vi "index_trigger.vi"(10 "fifo-counter":i32) -> (2 "index trigger":bool)   [LabVIEW 2015]
panel:
  # "(Ignoring the first iteration) This subvi returns true when the previous value \npassed in does not equal the current value passed in."
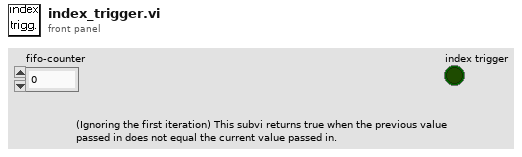
[diagram p1: front panel]
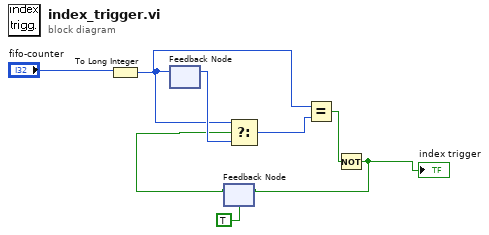
[diagram p0: block diagram]
diagram:
  n1 = To Long Integer(number="fifo-counter") -> (32bit integer=w6:i32)
  n2 = feedback #1() -> (w8:i32)  [unwired: 1 in]
  n3 = feedback-in #1(w6) -> ()
  n4 = feedback #2(TRUE) -> (w4:bool)
  n5 = Select(t=w6, s=w4, f=w8) -> (s? t:f=w7:i32)
  n6 = Equal?(x=w6, y=w7) -> (x = y?=w5:bool)
  n7 = Not(x=w5) -> (.not. x?=w1:bool)
  "index trigger" <- w1
  n8 = feedback-in #2(w1) -> ()
